vi "configure CONFIG array.vi"() -> (0 "CONFIG":T1(array[cluster]))   [LabVIEW 2011]
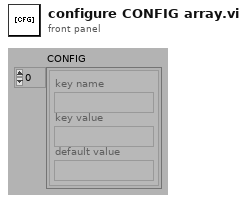
[diagram p1: front panel]
types:
  T1 = cluster{"key name":string, "key value":string, "default value":string}[]
  T2 = cluster{"name or relative path":string, string, string}
  T3 = cluster{"name or relative path":string, "Config Value":string, string}
  T4 = cluster{"name or relative path":string, "Config Value":string, "name or relative path":string}
  T5 = cluster{"key":string, "Config Value":string, string}
  T6 = cluster{"key":string, "Config Value":string, "name or relative path":string}
  T7 = cluster{"key":string, "Config Value":string, "name or relative path":string}[]
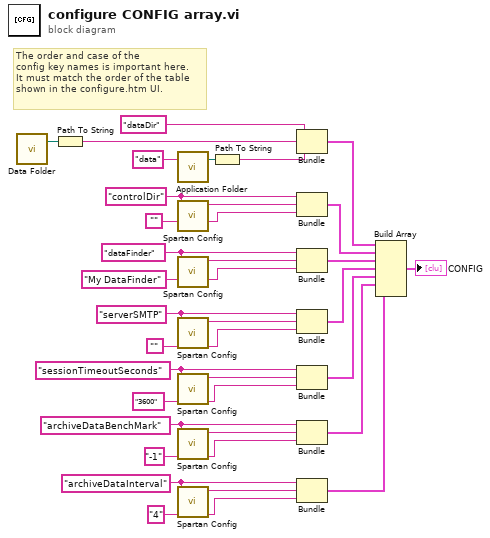
[diagram p0: block diagram]
diagram:
  w3 = "4" ("name or relative path")
  w5 = "archiveDataInterval" ("key")
  w8 = "-1" ("name or relative path")
  w6 = "archiveDataBenchMark" ("key")
  w9 = "3600" ("name or relative path")
  w11 = ""
  w28 = "controlDir" ("name or relative path")
  w21 = "sessionTimeoutSeconds" ("key")
  w27 = "dataFinder" ("name or relative path")
  w24 = "serverSMTP" ("key")
  w22 = ""
  w25 = "My DataFinder" ("name or relative path")
  # "The order and case of the\nconfig key names is important here.\nIt must match the order of the table\nshown in the configure.htm UI."
  n1 = call "Data Folder.vi"() -> ("Data Folder"=w32:path)  [unwired: 3 in]
  n2 = Path To String(path=w32) -> (string=w12:string)
  n3 = call "Application Folder.vi"("Relative Path (\"\" - Folder)"="data" ("name or relative path")) -> ("Application Folder"=w31:path)  [unwired: 2 in]
  n4 = call "Spartan Config.vi"("Default Value (\"\")"=w11, "Config Key (\"\")"=w28) -> ("Config Value"=w13:string)  [unwired: 7 in, 2 out]
  n5 = call "Spartan Config.vi"("Default Value (\"\")"=w25, "Config Key (\"\")"=w27) -> ("Config Value"=w26:string)  [unwired: 7 in, 2 out]
  n6 = call "Spartan Config.vi"("Default Value (\"\")"=w22, "Config Key (\"\")"=w24) -> ("Config Value"=w23:string)  [unwired: 7 in, 2 out]
  n7 = call "Spartan Config.vi"("Default Value (\"\")"=w9, "Config Key (\"\")"=w21) -> ("Config Value"=w20:string)  [unwired: 7 in, 2 out]
  n8 = call "Spartan Config.vi"("Default Value (\"\")"=w8, "Config Key (\"\")"=w6) -> ("Config Value"=w7:string)  [unwired: 7 in, 2 out]
  n9 = call "Spartan Config.vi"("Default Value (\"\")"=w3, "Config Key (\"\")"=w5) -> ("Config Value"=w4:string)  [unwired: 7 in, 2 out]
  n10 = Path To String(path=w31) -> (string=w14:string)
  n11 = Bundle("name or relative path"="dataDir", w12, w14) -> (w19:T2)  [unwired: 1 in]
  n12 = Bundle("name or relative path"=w28, "Config Value"=w13, w11) -> (w10:T3)  [unwired: 1 in]
  n13 = Bundle("name or relative path"=w27, "Config Value"=w26, "name or relative path"=w25) -> (w18:T4)  [unwired: 1 in]
  n14 = Bundle("key"=w24, "Config Value"=w23, w22) -> (w17:T5)  [unwired: 1 in]
  n15 = Bundle("key"=w21, "Config Value"=w20, "name or relative path"=w9) -> (w16:T6)  [unwired: 1 in]
  n16 = Bundle("key"=w6, "Config Value"=w7, "name or relative path"=w8) -> (w2:T6)  [unwired: 1 in]
  n17 = Bundle("key"=w5, "Config Value"=w4, "name or relative path"=w3) -> (w1:T6)  [unwired: 1 in]
  n18 = Build Array(w19, w10, w18, w17, w16, w2, w1) -> (→"CONFIG":T7)
